vi "释放通道.vi"(9 "通道":string, 11 "TCP Network Connection in":refnum<k5>) -> (0 "error out":errorcluster, 1 "ack":string, 3 "TCP Network Connection out":refnum<k5>)   [LabVIEW 2015]
uses:
  Global/SeverGlobal.vi
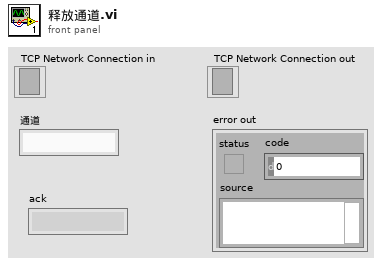
[diagram p1: front panel]
types:
  T1 = typedef "响应消息头.ctl" = string
  T2 = cluster{"TCP Ref":refnum<k5>, "A":u16, "COM":u16}
  T3 = cluster{"TCP Ref":refnum<k5>, "IN":u16, "OUT":u16}
  T4 = cluster{"TCP Ref":refnum<k5>, "Broadcast":refnum<k5>, "TF Ref":refnum<k5>, "IP":string, "port":u16, "userName":string, "passWord":string, "authority":string}[]
  T5 = cluster{"TCP Ref":refnum<k5>, "IP":string, "userName":string, "A":u16, "COM":u16, "time":u32}[]
  T6 = cluster{"TCP Ref":refnum<k5>, "IP":string, "userName":string, "IN":u16, "OUT":u16, "time":u32}[]
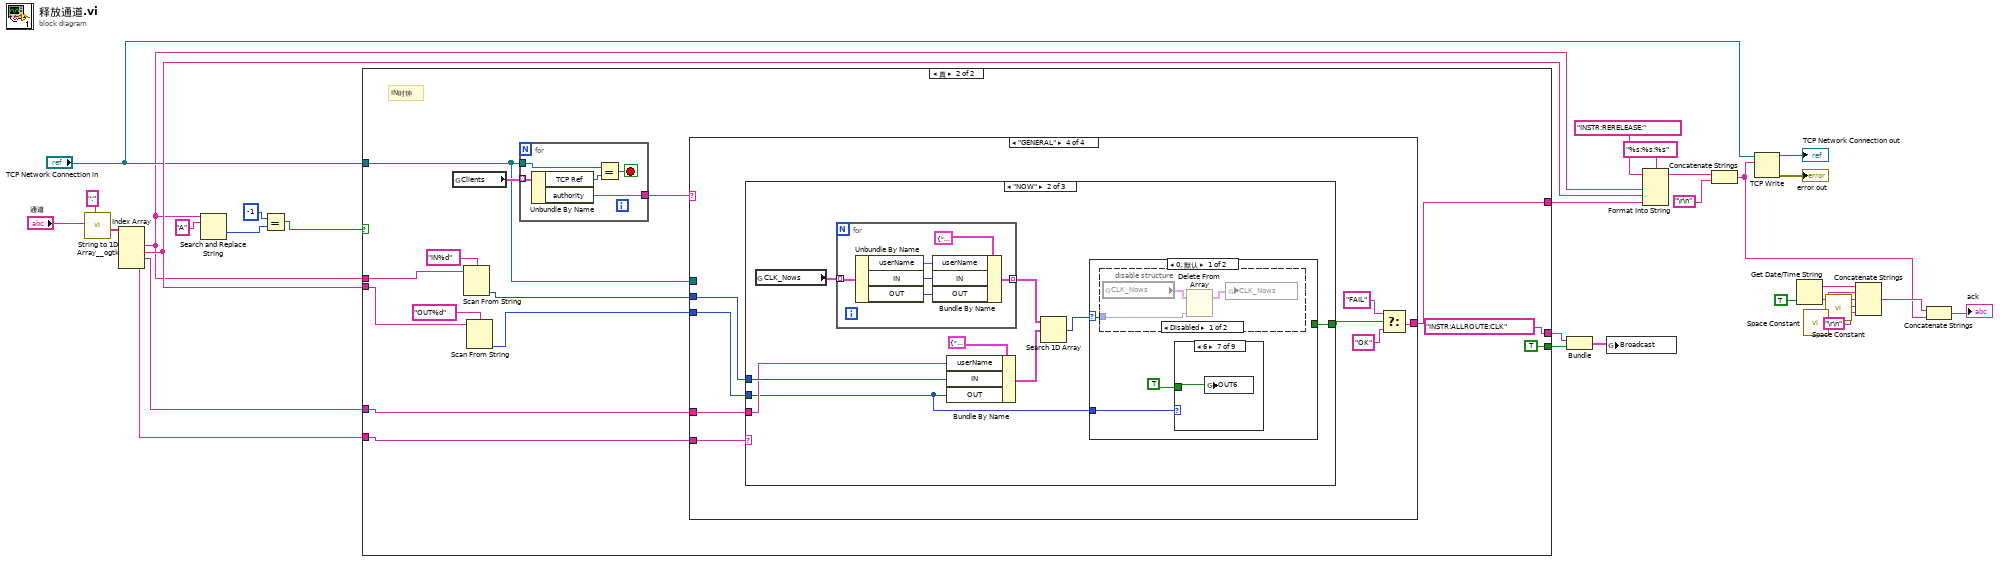
[diagram p0: block diagram]
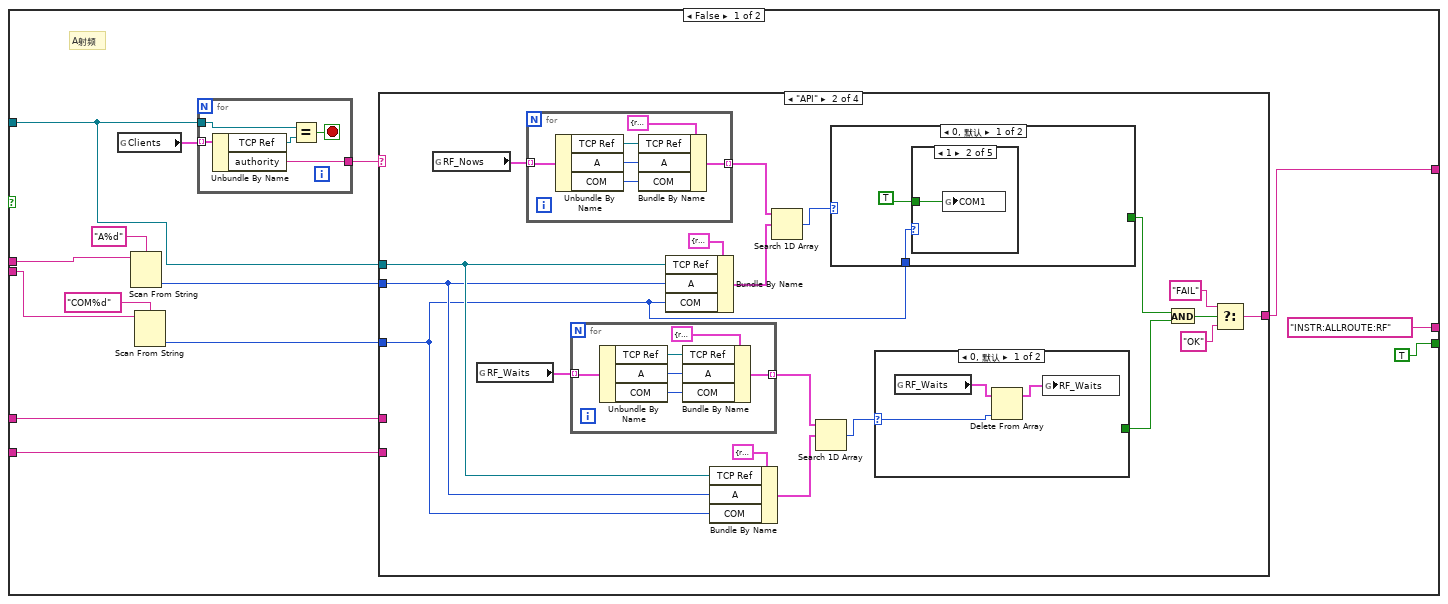
[diagram p2: hidden frame]
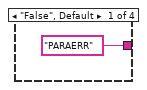
[diagram p3: hidden frame]
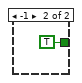
[diagram p4: hidden frame]
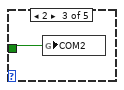
[diagram p6: hidden frame]
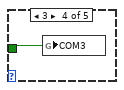
[diagram p7: hidden frame]
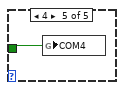
[diagram p8: hidden frame]
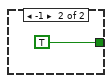
[diagram p9: hidden frame]
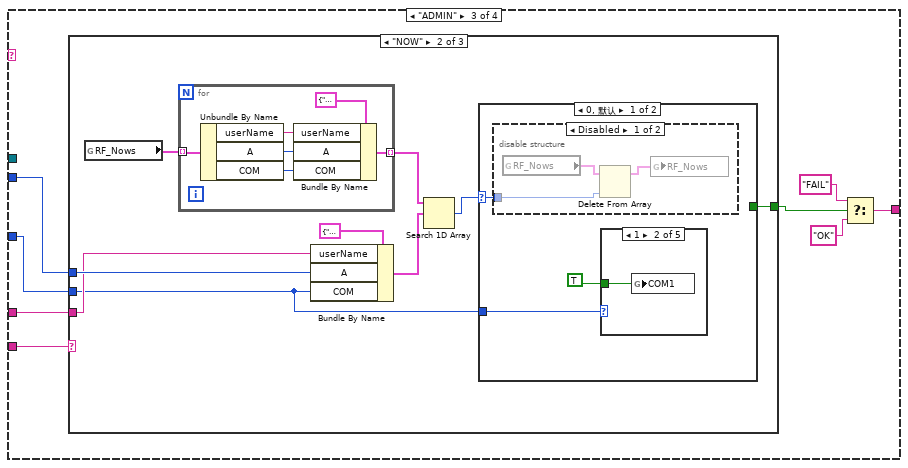
[diagram p10: hidden frame]
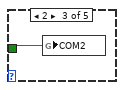
[diagram p14: hidden frame]
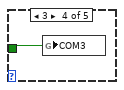
[diagram p15: hidden frame]
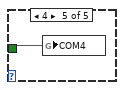
[diagram p16: hidden frame]
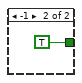
[diagram p17: hidden frame]
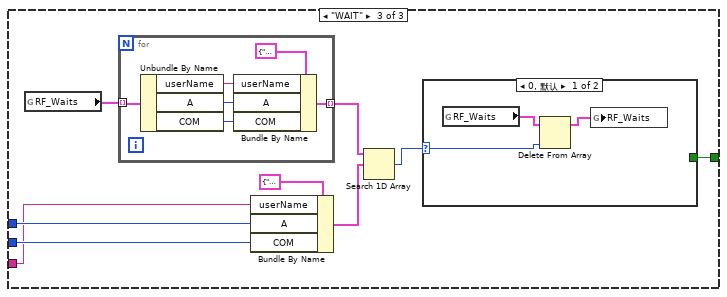
[diagram p18: hidden frame]
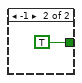
[diagram p19: hidden frame]
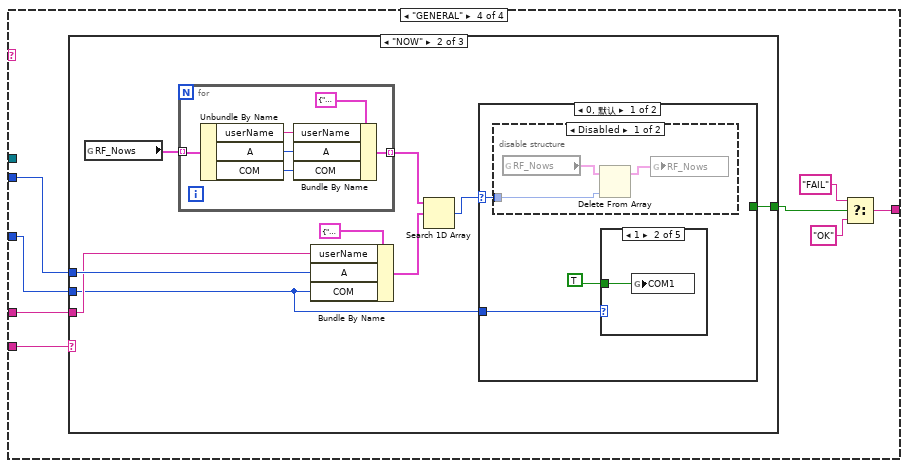
[diagram p20: hidden frame]
diagram:
  n1 = call <userlib>:"String to 1D Array__ogtk.vi"("delimiter (Tab)"=":", "string"="通道") -> ("Array of Strings"=w23:string[])  [unwired: 9 in]
  n2 = Index Array(array=w23) -> (element #1=w20:string, element #2=w31:string, element #3=w15:string, element #4=w14:string)  [unwired: 4 in]
  n3 = Search and Replace String(input string=w20, search string="A") -> (offset past replacement=w18:i32)  [unwired: 6 in, 3 out]
  n4 = Equal?(x=-1, y=w18) -> (x = y?=w16:bool)
  n5 = case shown="真" w16 {
    tunnel: w31 -> [w45 w213]
    tunnel: w20 -> [w44 w212]
    tunnel: [w37 w204] -> w13
    tunnel: "TCP Network Connection in" -> [w34 w207]
    tunnel: w15 -> [w36 w203]
    tunnel: w14 -> [w35 w202]
    tunnel: ["INSTR:ALLROUTE:RF" ("format string") "INSTR:ALLROUTE:CLK" ("format string")] -> w11
    tunnel: [TRUE TRUE] -> w10
    frame False {
      # "A射频"
      n6 = global read "SeverGlobal.vi" "Clients"() -> (w41:T4)
      n7 = Scan From String(format string="A%d", input string=w44) -> (output 1=w39:i32)  [unwired: 3 in, 3 out]
      n8 = Scan From String(format string="COM%d", input string=w45) -> (output 1=w38:i32)  [unwired: 3 in, 3 out]
      n9 = for {
        tunnel: w41 -> [w199] mode=indexing
        tunnel: w34 -> [w197]
        tunnel: [w195] -> w40
        stop <- w196 stop-if-true
        n10 = Unbundle By Name(w199) -> ("TCP Ref"=w198:refnum<k5>, "authority"=w195:string)
        n11 = Equal?(x=w197, y=w198) -> (x = y?=w196:bool)
      }
      n12 = case shown="\"API\"" w40 {
        tunnel: w34 -> [_ w55 _ _]
        tunnel: w39 -> [_ w54 w96 w149]
        tunnel: w38 -> [_ w47 w95 w148]
        tunnel: ["PARAERR" ("format string") w48 w92 w145] -> w37
        tunnel: w36 -> [_ _ w91 w144]
        tunnel: w35 -> [_ _ w90 w143]
        frame "False", Default {
        }
        frame "API" {
          n13 = global read "SeverGlobal.vi" "RF_Nows"() -> (w65:T5)
          n14 = global read "SeverGlobal.vi" "RF_Waits"() -> (w56:T5)
          n15 = for {
            tunnel: w65 -> [w88] mode=indexing
            tunnel: [w83] -> w63 mode=indexing
            n16 = Unbundle By Name(w88) -> ("TCP Ref"=w85:refnum<k5>, "A"=w86:u16, "COM"=w84:u16)
            n17 = Bundle By Name(cluster=T2 {"TCP Ref"=refnum, "A"=0, "COM"=0} ("RF_Now"), "TCP Ref"=w85, "A"=w86, "COM"=w84) -> (w83:T2)
          }
          n18 = for {
            tunnel: w56 -> [w75] mode=indexing
            tunnel: [w70] -> w58 mode=indexing
            n19 = Unbundle By Name(w75) -> ("TCP Ref"=w72:refnum<k5>, "A"=w73:u16, "COM"=w71:u16)
            n20 = Bundle By Name(cluster=T2 {"TCP Ref"=refnum, "A"=0, "COM"=0} ("RF_Now"), "TCP Ref"=w72, "A"=w73, "COM"=w71) -> (w70:T2)
          }
          n21 = Bundle By Name(cluster=T2 {"TCP Ref"=refnum, "A"=0, "COM"=0} ("RF_Now"), "TCP Ref"=w55, "A"=w54, "COM"=w47) -> (w62:T2)
          n22 = Bundle By Name(cluster=T2 {"TCP Ref"=refnum, "A"=0, "COM"=0} ("RF_Now"), "TCP Ref"=w55, "A"=w54, "COM"=w47) -> (w59:T2)
          n23 = Search 1D Array(1D array=w63, element=w62) -> (index of element=w61:i32)  [unwired: 1 in]
          n24 = Search 1D Array(1D array=w58, element=w59) -> (index of element=w60:i32)  [unwired: 1 in]
          n25 = case shown="0, 默认" w61 {
            tunnel: [_ TRUE] -> w53
            tunnel: w47 -> [w76 _]
            frame 0, Default {
              n26 = case shown="1" w76 {
                tunnel: TRUE ("COM1") -> [_ w78 w79 w80 w81]
                frame 0, Default {
                }
                frame 1 {
                  n27 = global write "SeverGlobal.vi" "COM1"(w78) -> ()
                }
                frame 2 {
                  n28 = global write "SeverGlobal.vi" "COM2"(w79) -> ()
                }
                frame 3 {
                  n29 = global write "SeverGlobal.vi" "COM3"(w80) -> ()
                }
                frame 4 {
                  n30 = global write "SeverGlobal.vi" "COM4"(w81) -> ()
                }
              }
            }
            frame -1 {
            }
          }
          n31 = case shown="0, 默认" w60 {
            selector: w60 -> [w67 _]
            tunnel: [_ TRUE] -> w52
            frame 0, Default {
              n32 = global read "SeverGlobal.vi" "RF_Waits"() -> (w68:T5)
              n33 = Delete From Array(array=w68, index=w67) -> (array with subset deleted=w66:T5)  [unwired: 1 in, 1 out]
              n34 = global write "SeverGlobal.vi" "RF_Waits"(w66) -> ()
            }
            frame -1 {
            }
          }
          n35 = And(x=w53, y=w52) -> (x .and. y?=w51:bool)
          n36 = Select(t="FAIL" ("format string"), s=w51, f="OK" ("format string")) -> (s? t:f=w48:string)
        }
        frame "ADMIN" {
          n37 = case shown="\"NOW\"" w90 {
            tunnel: w96 -> [_ w101 w127]
            tunnel: w95 -> [_ w97 w126]
            tunnel: [_ w100 w125] -> w89
            tunnel: w91 -> [_ w98 w123]
            frame Default {
            }
            frame "NOW" {
              n38 = global read "SeverGlobal.vi" "RF_Nows"() -> (w105:T5)
              n39 = for {
                tunnel: w105 -> [w122] mode=indexing
                tunnel: [w118] -> w104 mode=indexing
                n40 = Unbundle By Name(w122) -> ("userName"=w120:string, "A"=w121:u16, "COM"=w119:u16)
                n41 = Bundle By Name(cluster=cluster{"userName":string, "A":u16, "COM":u16} {"userName"="", "A"=0, "COM"=0} ("RF_Now"), "userName"=w120, "A"=w121, "COM"=w119) -> (w118:cluster{"userName":string, "A":u16, "COM":u16})
              }
              n42 = Bundle By Name(cluster=cluster{"userName":string, "A":u16, "COM":u16} {"userName"="", "A"=0, "COM"=0} ("RF_Now"), "userName"=w98, "A"=w101, "COM"=w97) -> (w103:cluster{"userName":string, "A":u16, "COM":u16})
              n43 = Search 1D Array(1D array=w104, element=w103) -> (index of element=w102:i32)  [unwired: 1 in]
              n44 = case shown="0, 默认" w102 {
                selector: w102 -> [w108 _]
                tunnel: [_ TRUE] -> w100
                tunnel: w97 -> [w107 _]
                frame 0, Default {
                  n45 = disable-structure shown="Disabled" {
                    disable-tunnel: w108 -> [w110 _]
                    frame Disabled {
                      n46 = global read "SeverGlobal.vi" "RF_Nows"() -> (w111:T5)
                      n47 = Delete From Array(array=w111, index=w110) -> (array with subset deleted=w109:T5)  [unwired: 1 in, 1 out]
                      n48 = global write "SeverGlobal.vi" "RF_Nows"(w109) -> ()
                    }
                    frame Enabled {
                    }
                  }
                  n49 = case shown="1" w107 {
                    tunnel: TRUE ("COM1") -> [_ w112 w113 w114 w115]
                    frame 0, Default {
                    }
                    frame 1 {
                      n50 = global write "SeverGlobal.vi" "COM1"(w112) -> ()
                    }
                    frame 2 {
                      n51 = global write "SeverGlobal.vi" "COM2"(w113) -> ()
                    }
                    frame 3 {
                      n52 = global write "SeverGlobal.vi" "COM3"(w114) -> ()
                    }
                    frame 4 {
                      n53 = global write "SeverGlobal.vi" "COM4"(w115) -> ()
                    }
                  }
                }
                frame -1 {
                }
              }
            }
            frame "WAIT" {
              n54 = global read "SeverGlobal.vi" "RF_Waits"() -> (w131:T5)
              n55 = for {
                tunnel: w131 -> [w141] mode=indexing
                tunnel: [w137] -> w130 mode=indexing
                n56 = Unbundle By Name(w141) -> ("userName"=w139:string, "A"=w140:u16, "COM"=w138:u16)
                n57 = Bundle By Name(cluster=cluster{"userName":string, "A":u16, "COM":u16} {"userName"="", "A"=0, "COM"=0} ("RF_Now"), "userName"=w139, "A"=w140, "COM"=w138) -> (w137:cluster{"userName":string, "A":u16, "COM":u16})
              }
              n58 = Bundle By Name(cluster=cluster{"userName":string, "A":u16, "COM":u16} {"userName"="", "A"=0, "COM"=0} ("RF_Now"), "userName"=w123, "A"=w127, "COM"=w126) -> (w129:cluster{"userName":string, "A":u16, "COM":u16})
              n59 = Search 1D Array(1D array=w130, element=w129) -> (index of element=w128:i32)  [unwired: 1 in]
              n60 = case shown="0, 默认" w128 {
                selector: w128 -> [w133 _]
                tunnel: [_ TRUE] -> w125
                frame 0, Default {
                  n61 = global read "SeverGlobal.vi" "RF_Waits"() -> (w134:T5)
                  n62 = Delete From Array(array=w134, index=w133) -> (array with subset deleted=w132:T5)  [unwired: 1 in, 1 out]
                  n63 = global write "SeverGlobal.vi" "RF_Waits"(w132) -> ()
                }
                frame -1 {
                }
              }
            }
          }
          n64 = Select(t="FAIL" ("format string"), s=w89, f="OK" ("format string")) -> (s? t:f=w92:string)
        }
        frame "GENERAL" {
          n65 = case shown="\"NOW\"" w143 {
            tunnel: w149 -> [_ w154 w180]
            tunnel: w148 -> [_ w150 w179]
            tunnel: [_ w153 w178] -> w142
            tunnel: w144 -> [_ w151 w176]
            frame Default {
            }
            frame "NOW" {
              n66 = global read "SeverGlobal.vi" "RF_Nows"() -> (w158:T5)
              n67 = for {
                tunnel: w158 -> [w175] mode=indexing
                tunnel: [w171] -> w157 mode=indexing
                n68 = Unbundle By Name(w175) -> ("userName"=w173:string, "A"=w174:u16, "COM"=w172:u16)
                n69 = Bundle By Name(cluster=cluster{"userName":string, "A":u16, "COM":u16} {"userName"="", "A"=0, "COM"=0} ("RF_Now"), "userName"=w173, "A"=w174, "COM"=w172) -> (w171:cluster{"userName":string, "A":u16, "COM":u16})
              }
              n70 = Bundle By Name(cluster=cluster{"userName":string, "A":u16, "COM":u16} {"userName"="", "A"=0, "COM"=0} ("RF_Now"), "userName"=w151, "A"=w154, "COM"=w150) -> (w156:cluster{"userName":string, "A":u16, "COM":u16})
              n71 = Search 1D Array(1D array=w157, element=w156) -> (index of element=w155:i32)  [unwired: 1 in]
              n72 = case shown="0, 默认" w155 {
                selector: w155 -> [w161 _]
                tunnel: [_ TRUE] -> w153
                tunnel: w150 -> [w160 _]
                frame 0, Default {
                  n73 = disable-structure shown="Disabled" {
                    disable-tunnel: w161 -> [w163 _]
                    frame Disabled {
                      n74 = global read "SeverGlobal.vi" "RF_Nows"() -> (w164:T5)
                      n75 = Delete From Array(array=w164, index=w163) -> (array with subset deleted=w162:T5)  [unwired: 1 in, 1 out]
                      n76 = global write "SeverGlobal.vi" "RF_Nows"(w162) -> ()
                    }
                    frame Enabled {
                    }
                  }
                  n77 = case shown="1" w160 {
                    tunnel: TRUE ("COM1") -> [_ w165 w166 w167 w168]
                    frame 0, Default {
                    }
                    frame 1 {
                      n78 = global write "SeverGlobal.vi" "COM1"(w165) -> ()
                    }
                    frame 2 {
                      n79 = global write "SeverGlobal.vi" "COM2"(w166) -> ()
                    }
                    frame 3 {
                      n80 = global write "SeverGlobal.vi" "COM3"(w167) -> ()
                    }
                    frame 4 {
                      n81 = global write "SeverGlobal.vi" "COM4"(w168) -> ()
                    }
                  }
                }
                frame -1 {
                }
              }
            }
            frame "WAIT" {
              n82 = global read "SeverGlobal.vi" "RF_Waits"() -> (w184:T5)
              n83 = for {
                tunnel: w184 -> [w194] mode=indexing
                tunnel: [w190] -> w183 mode=indexing
                n84 = Unbundle By Name(w194) -> ("userName"=w192:string, "A"=w193:u16, "COM"=w191:u16)
                n85 = Bundle By Name(cluster=cluster{"userName":string, "A":u16, "COM":u16} {"userName"="", "A"=0, "COM"=0} ("RF_Now"), "userName"=w192, "A"=w193, "COM"=w191) -> (w190:cluster{"userName":string, "A":u16, "COM":u16})
              }
              n86 = Bundle By Name(cluster=cluster{"userName":string, "A":u16, "COM":u16} {"userName"="", "A"=0, "COM"=0} ("RF_Now"), "userName"=w176, "A"=w180, "COM"=w179) -> (w182:cluster{"userName":string, "A":u16, "COM":u16})
              n87 = Search 1D Array(1D array=w183, element=w182) -> (index of element=w181:i32)  [unwired: 1 in]
              n88 = case shown="0, 默认" w181 {
                selector: w181 -> [w186 _]
                tunnel: [_ TRUE] -> w178
                frame 0, Default {
                  n89 = global read "SeverGlobal.vi" "RF_Waits"() -> (w187:T5)
                  n90 = Delete From Array(array=w187, index=w186) -> (array with subset deleted=w185:T5)  [unwired: 1 in, 1 out]
                  n91 = global write "SeverGlobal.vi" "RF_Waits"(w185) -> ()
                }
                frame -1 {
                }
              }
            }
          }
          n92 = Select(t="FAIL" ("format string"), s=w142, f="OK" ("format string")) -> (s? t:f=w145:string)
        }
      }
    }
    frame True {
      # "IN时钟"
      n93 = global read "SeverGlobal.vi" "Clients"() -> (w209:T4)
      n94 = Scan From String(format string="IN%d", input string=w212) -> (output 1=w206:i32)  [unwired: 3 in, 3 out]
      n95 = Scan From String(format string="OUT%d", input string=w213) -> (output 1=w205:i32)  [unwired: 3 in, 3 out]
      n96 = for {
        tunnel: w209 -> [w379] mode=indexing
        tunnel: w207 -> [w377]
        tunnel: [w375] -> w208
        stop <- w376 stop-if-true
        n97 = Unbundle By Name(w379) -> ("TCP Ref"=w378:refnum<k5>, "authority"=w375:string)
        n98 = Equal?(x=w377, y=w378) -> (x = y?=w376:bool)
      }
      n99 = case shown="\"GENERAL\"" w208 {
        tunnel: w207 -> [_ w225 _ _]
        tunnel: w206 -> [_ w224 w268 w325]
        tunnel: w205 -> [_ w215 w267 w324]
        tunnel: ["PARAERR" ("format string") w218 w261 w318] -> w204
        tunnel: w203 -> [_ _ w266 w323]
        tunnel: w202 -> [_ _ w265 w322]
        frame "False", Default {
        }
        frame "API" {
          n100 = global read "SeverGlobal.vi" "CLK_Nows"() -> (w233:T6)
          n101 = global read "SeverGlobal.vi" "CLK_Waits"() -> (w226:T6)
          n102 = for {
            tunnel: w233 -> [w260] mode=indexing
            tunnel: [w256] -> w232 mode=indexing
            n103 = Unbundle By Name(w260) -> ("TCP Ref"=w258:refnum<k5>, "IN"=w259:u16, "OUT"=w257:u16)
            n104 = Bundle By Name(cluster=T3 {"TCP Ref"=refnum, "IN"=0, "OUT"=0} ("RF_Now"), "TCP Ref"=w258, "IN"=w259, "OUT"=w257) -> (w256:T3)
          }
          n105 = for {
            tunnel: w226 -> [w243] mode=indexing
            tunnel: [w239] -> w227 mode=indexing
            n106 = Unbundle By Name(w243) -> ("TCP Ref"=w241:refnum<k5>, "IN"=w242:u16, "OUT"=w240:u16)
            n107 = Bundle By Name(cluster=T3 {"TCP Ref"=refnum, "IN"=0, "OUT"=0} ("RF_Now"), "TCP Ref"=w241, "IN"=w242, "OUT"=w240) -> (w239:T3)
          }
          n108 = Bundle By Name(cluster=T3 {"TCP Ref"=refnum, "IN"=0, "OUT"=0} ("RF_Now"), "TCP Ref"=w225, "IN"=w224, "OUT"=w215) -> (w231:T3)
          n109 = Bundle By Name(cluster=T3 {"TCP Ref"=refnum, "IN"=0, "OUT"=0} ("RF_Now"), "TCP Ref"=w225, "IN"=w224, "OUT"=w215) -> (w228:T3)
          n110 = Search 1D Array(1D array=w232, element=w231) -> (index of element=w230:i32)  [unwired: 1 in]
          n111 = Search 1D Array(1D array=w227, element=w228) -> (index of element=w229:i32)  [unwired: 1 in]
          n112 = case shown="0, 默认" w230 {
            tunnel: [_ TRUE] -> w223
            tunnel: w215 -> [w244 _]
            frame 0, Default {
              n113 = case shown="1" w244 {
                tunnel: TRUE ("COM1") -> [_ w246 w247 w248 w249 w250 w251 w252 w253]
                frame 0, Default {
                }
                frame 1 {
                  n114 = global write "SeverGlobal.vi" "OUT1"(w246) -> ()
                }
                frame 2 {
                  n115 = global write "SeverGlobal.vi" "OUT2"(w247) -> ()
                }
                frame 3 {
                  n116 = global write "SeverGlobal.vi" "OUT3"(w248) -> ()
                }
                frame 4 {
                  n117 = global write "SeverGlobal.vi" "OUT4"(w249) -> ()
                }
                frame 5 {
                  n118 = global write "SeverGlobal.vi" "OUT5"(w250) -> ()
                }
                frame 6 {
                  n119 = global write "SeverGlobal.vi" "OUT6"(w251) -> ()
                }
                frame 7 {
                  n120 = global write "SeverGlobal.vi" "OUT7"(w252) -> ()
                }
                frame 8 {
                  n121 = global write "SeverGlobal.vi" "OUT8"(w253) -> ()
                }
              }
            }
            frame -1 {
            }
          }
          n122 = case shown="0, 默认" w229 {
            selector: w229 -> [w235 _]
            tunnel: [_ TRUE] -> w222
            frame 0, Default {
              n123 = global read "SeverGlobal.vi" "CLK_Waits"() -> (w236:T6)
              n124 = Delete From Array(array=w236, index=w235) -> (array with subset deleted=w234:T6)  [unwired: 1 in, 1 out]
              n125 = global write "SeverGlobal.vi" "CLK_Waits"(w234) -> ()
            }
            frame -1 {
            }
          }
          n126 = And(x=w223, y=w222) -> (x .and. y?=w221:bool)
          n127 = Select(t="FAIL" ("format string"), s=w221, f="OK" ("format string")) -> (s? t:f=w218:string)
        }
        frame "ADMIN" {
          n128 = case shown="\"NOW\"" w265 {
            tunnel: w268 -> [_ w273 w303]
            tunnel: w267 -> [_ w269 w302]
            tunnel: [_ w272 w301] -> w262
            tunnel: w266 -> [_ w271 w299]
            frame Default {
            }
            frame "NOW" {
              n129 = global read "SeverGlobal.vi" "CLK_Nows"() -> (w277:T6)
              n130 = for {
                tunnel: w277 -> [w298] mode=indexing
                tunnel: [w294] -> w276 mode=indexing
                n131 = Unbundle By Name(w298) -> ("userName"=w296:string, "IN"=w297:u16, "OUT"=w295:u16)
                n132 = Bundle By Name(cluster=cluster{"userName":string, "IN":u16, "OUT":u16} {"userName"="", "IN"=0, "OUT"=0} ("RF_Now"), "userName"=w296, "IN"=w297, "OUT"=w295) -> (w294:cluster{"userName":string, "IN":u16, "OUT":u16})
              }
              n133 = Bundle By Name(cluster=cluster{"userName":string, "IN":u16, "OUT":u16} {"userName"="", "IN"=0, "OUT"=0} ("RF_Now"), "userName"=w271, "IN"=w273, "OUT"=w269) -> (w275:cluster{"userName":string, "IN":u16, "OUT":u16})
              n134 = Search 1D Array(1D array=w276, element=w275) -> (index of element=w274:i32)  [unwired: 1 in]
              n135 = case shown="0, 默认" w274 {
                selector: w274 -> [w280 _]
                tunnel: [_ TRUE] -> w272
                tunnel: w269 -> [w278 _]
                frame 0, Default {
                  n136 = disable-structure shown="Disabled" {
                    disable-tunnel: w280 -> [w290 _]
                    frame Disabled {
                      n137 = global read "SeverGlobal.vi" "CLK_Nows"() -> (w291:T6)
                      n138 = Delete From Array(array=w291, index=w290) -> (array with subset deleted=w289:T6)  [unwired: 1 in, 1 out]
                      n139 = global write "SeverGlobal.vi" "CLK_Nows"(w289) -> ()
                    }
                    frame Enabled {
                    }
                  }
                  n140 = case shown="1" w278 {
                    tunnel: TRUE ("COM1") -> [_ w281 w282 w283 w284 w285 w286 w287 w288]
                    frame 0, Default {
                    }
                    frame 1 {
                      n141 = global write "SeverGlobal.vi" "OUT1"(w281) -> ()
                    }
                    frame 2 {
                      n142 = global write "SeverGlobal.vi" "OUT2"(w282) -> ()
                    }
                    frame 3 {
                      n143 = global write "SeverGlobal.vi" "OUT3"(w283) -> ()
                    }
                    frame 4 {
                      n144 = global write "SeverGlobal.vi" "OUT4"(w284) -> ()
                    }
                    frame 5 {
                      n145 = global write "SeverGlobal.vi" "OUT5"(w285) -> ()
                    }
                    frame 6 {
                      n146 = global write "SeverGlobal.vi" "OUT6"(w286) -> ()
                    }
                    frame 7 {
                      n147 = global write "SeverGlobal.vi" "OUT7"(w287) -> ()
                    }
                    frame 8 {
                      n148 = global write "SeverGlobal.vi" "OUT8"(w288) -> ()
                    }
                  }
                }
                frame -1 {
                }
              }
            }
            frame "WAIT" {
              n149 = global read "SeverGlobal.vi" "CLK_Waits"() -> (w307:T6)
              n150 = for {
                tunnel: w307 -> [w317] mode=indexing
                tunnel: [w313] -> w306 mode=indexing
                n151 = Unbundle By Name(w317) -> ("userName"=w315:string, "IN"=w316:u16, "OUT"=w314:u16)
                n152 = Bundle By Name(cluster=cluster{"userName":string, "A":u16, "COM":u16} {"userName"="", "A"=0, "COM"=0} ("RF_Now"), "userName"=w315, "A"=w316, "COM"=w314) -> (w313:cluster{"userName":string, "A":u16, "COM":u16})
              }
              n153 = Bundle By Name(cluster=cluster{"userName":string, "A":u16, "COM":u16} {"userName"="", "A"=0, "COM"=0} ("RF_Now"), "userName"=w299, "A"=w303, "COM"=w302) -> (w305:cluster{"userName":string, "A":u16, "COM":u16})
              n154 = Search 1D Array(1D array=w306, element=w305) -> (index of element=w304:i32)  [unwired: 1 in]
              n155 = case shown="0, 默认" w304 {
                selector: w304 -> [w309 _]
                tunnel: [_ TRUE] -> w301
                frame 0, Default {
                  n156 = global read "SeverGlobal.vi" "CLK_Waits"() -> (w310:T6)
                  n157 = Delete From Array(array=w310, index=w309) -> (array with subset deleted=w308:T6)  [unwired: 1 in, 1 out]
                  n158 = global write "SeverGlobal.vi" "CLK_Waits"(w308) -> ()
                }
                frame -1 {
                }
              }
            }
          }
          n159 = Select(t="FAIL" ("format string"), s=w262, f="OK" ("format string")) -> (s? t:f=w261:string)
        }
        frame "GENERAL" {
          n160 = case shown="\"NOW\"" w322 {
            tunnel: w325 -> [_ w330 w360]
            tunnel: w324 -> [_ w326 w359]
            tunnel: [_ w329 w358] -> w319
            tunnel: w323 -> [_ w328 w356]
            frame Default {
            }
            frame "NOW" {
              n161 = global read "SeverGlobal.vi" "CLK_Nows"() -> (w334:T6)
              n162 = for {
                tunnel: w334 -> [w355] mode=indexing
                tunnel: [w351] -> w333 mode=indexing
                n163 = Unbundle By Name(w355) -> ("userName"=w353:string, "IN"=w354:u16, "OUT"=w352:u16)
                n164 = Bundle By Name(cluster=cluster{"userName":string, "IN":u16, "OUT":u16} {"userName"="", "IN"=0, "OUT"=0} ("RF_Now"), "userName"=w353, "IN"=w354, "OUT"=w352) -> (w351:cluster{"userName":string, "IN":u16, "OUT":u16})
              }
              n165 = Bundle By Name(cluster=cluster{"userName":string, "IN":u16, "OUT":u16} {"userName"="", "IN"=0, "OUT"=0} ("RF_Now"), "userName"=w328, "IN"=w330, "OUT"=w326) -> (w332:cluster{"userName":string, "IN":u16, "OUT":u16})
              n166 = Search 1D Array(1D array=w333, element=w332) -> (index of element=w331:i32)  [unwired: 1 in]
              n167 = case shown="0, 默认" w331 {
                selector: w331 -> [w337 _]
                tunnel: [_ TRUE] -> w329
                tunnel: w326 -> [w335 _]
                frame 0, Default {
                  n168 = disable-structure shown="Disabled" {
                    disable-tunnel: w337 -> [w347 _]
                    frame Disabled {
                      n169 = global read "SeverGlobal.vi" "CLK_Nows"() -> (w348:T6)
                      n170 = Delete From Array(array=w348, index=w347) -> (array with subset deleted=w346:T6)  [unwired: 1 in, 1 out]
                      n171 = global write "SeverGlobal.vi" "CLK_Nows"(w346) -> ()
                    }
                    frame Enabled {
                    }
                  }
                  n172 = case shown="6" w335 {
                    tunnel: TRUE ("COM1") -> [_ w338 w339 w340 w341 w342 w343 w344 w345]
                    frame 0, Default {
                    }
                    frame 1 {
                      n173 = global write "SeverGlobal.vi" "OUT1"(w338) -> ()
                    }
                    frame 2 {
                      n174 = global write "SeverGlobal.vi" "OUT2"(w339) -> ()
                    }
                    frame 3 {
                      n175 = global write "SeverGlobal.vi" "OUT3"(w340) -> ()
                    }
                    frame 4 {
                      n176 = global write "SeverGlobal.vi" "OUT4"(w341) -> ()
                    }
                    frame 5 {
                      n177 = global write "SeverGlobal.vi" "OUT5"(w342) -> ()
                    }
                    frame 6 {
                      n178 = global write "SeverGlobal.vi" "OUT6"(w343) -> ()
                    }
                    frame 7 {
                      n179 = global write "SeverGlobal.vi" "OUT7"(w344) -> ()
                    }
                    frame 8 {
                      n180 = global write "SeverGlobal.vi" "OUT8"(w345) -> ()
                    }
                  }
                }
                frame -1 {
                }
              }
            }
            frame "WAIT" {
              n181 = global read "SeverGlobal.vi" "CLK_Waits"() -> (w364:T6)
              n182 = for {
                tunnel: w364 -> [w374] mode=indexing
                tunnel: [w370] -> w363 mode=indexing
                n183 = Unbundle By Name(w374) -> ("userName"=w372:string, "IN"=w373:u16, "OUT"=w371:u16)
                n184 = Bundle By Name(cluster=cluster{"userName":string, "A":u16, "COM":u16} {"userName"="", "A"=0, "COM"=0} ("RF_Now"), "userName"=w372, "A"=w373, "COM"=w371) -> (w370:cluster{"userName":string, "A":u16, "COM":u16})
              }
              n185 = Bundle By Name(cluster=cluster{"userName":string, "A":u16, "COM":u16} {"userName"="", "A"=0, "COM"=0} ("RF_Now"), "userName"=w356, "A"=w360, "COM"=w359) -> (w362:cluster{"userName":string, "A":u16, "COM":u16})
              n186 = Search 1D Array(1D array=w363, element=w362) -> (index of element=w361:i32)  [unwired: 1 in]
              n187 = case shown="0, 默认" w361 {
                selector: w361 -> [w366 _]
                tunnel: [_ TRUE] -> w358
                frame 0, Default {
                  n188 = global read "SeverGlobal.vi" "CLK_Waits"() -> (w367:T6)
                  n189 = Delete From Array(array=w367, index=w366) -> (array with subset deleted=w365:T6)  [unwired: 1 in, 1 out]
                  n190 = global write "SeverGlobal.vi" "CLK_Waits"(w365) -> ()
                }
                frame -1 {
                }
              }
            }
          }
          n191 = Select(t="FAIL" ("format string"), s=w319, f="OK" ("format string")) -> (s? t:f=w318:string)
        }
      }
    }
  }
  n192 = Bundle("format string"=w11, w10) -> (w12:cluster{"format string":string, bool})  [unwired: 1 in]
  n193 = global write "SeverGlobal.vi" "Broadcast"(w12) -> ()
  n194 = Format Into String(format string="%s:%s:%s", initial string=T1 "INSTR:RERELEASE:" ("Combo Box"), w20, w31, w13) -> (resulting string=w30:string)  [unwired: 1 in, 1 out]
  n195 = Concatenate Strings(w30, "\r\n") -> (w1:string)
  n196 = TCP Write(connection ID="TCP Network Connection in", data in=w1) -> (connection ID out=→"TCP Network Connection out":refnum<k5>, error out=→"error out":errorcluster)  [unwired: 2 in, 1 out]
  n197 = Get Date/Time String(want seconds? (F)=TRUE ("需要秒？(F)")) -> (date string=w4:string, time string=w5:string)  [unwired: 2 in]
  n198 = call <vilib>:"Space Constant.vi"() -> ("String"=w6:string)
  n199 = call <vilib>:"Space Constant.vi"() -> ("String"=w7:string)
  n200 = Concatenate Strings(w4, w6, w5, w7, "\r\n") -> (w9:string)
  n201 = Concatenate Strings(w9, w1) -> (→"ack":string)
